vi "move.vi"(10 "dist(mm)":dbl, 11 "Manual Positioning":T1) -> (3 "MoveString":string)   [LabVIEW 2022 SP3]
uses:
  MoveSwitch.ctl
panel:
  out "number":i32
  out "array":bool[](array[boolean])
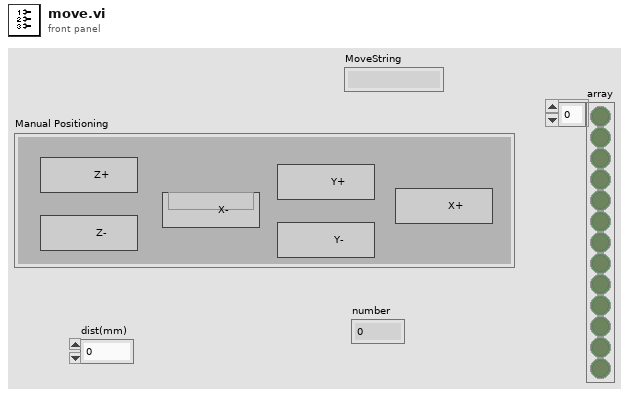
[diagram p1: front panel]
types:
  T1 = typedef "MoveSwitch.ctl" = cluster{"X+":bool, "X-":bool, "Y+":bool, "Y-":bool, "Z+":bool, "Z-":bool}
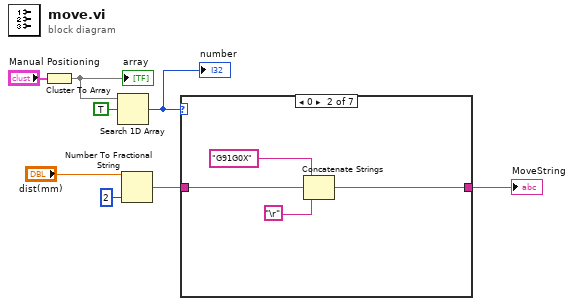
[diagram p0: block diagram]
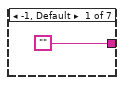
[diagram p2: hidden frame]
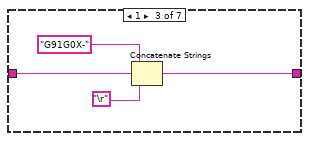
[diagram p3: hidden frame]
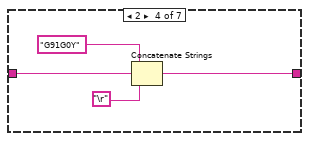
[diagram p4: hidden frame]
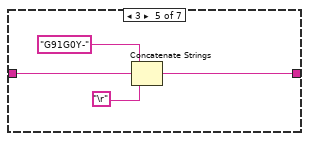
[diagram p5: hidden frame]
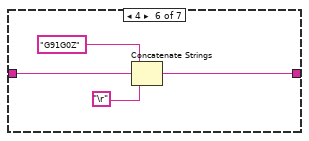
[diagram p6: hidden frame]
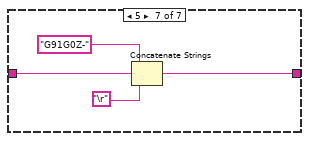
[diagram p7: hidden frame]
diagram:
  n1 = Cluster To Array(cluster="Manual Positioning") -> (array=w7:bool[])
  "array" <- w7
  n2 = Search 1D Array(1D array=w7, element=TRUE) -> (index of element=w5:i32)  [unwired: 1 in]
  "number" <- w5
  n3 = Number To Fractional String(number="dist(mm)", precision (6)=i16 2) -> (F-format string=w2:string)  [unwired: 2 in]
  n4 = case shown="0" w5 {
    tunnel: w2 -> [_ w12 w16 w20 w24 w28 w32]
    tunnel: ["" w10 w14 w18 w22 w26 w30] -> w1
    frame -1, Default {
    }
    frame 0 {
      n5 = Concatenate Strings("G91G0X", w12, "\r") -> (w10:string)
    }
    frame 1 {
      n6 = Concatenate Strings("G91G0X-", w16, "\r") -> (w14:string)
    }
    frame 2 {
      n7 = Concatenate Strings("G91G0Y", w20, "\r") -> (w18:string)
    }
    frame 3 {
      n8 = Concatenate Strings("G91G0Y-", w24, "\r") -> (w22:string)
    }
    frame 4 {
      n9 = Concatenate Strings("G91G0Z", w28, "\r") -> (w26:string)
    }
    frame 5 {
      n10 = Concatenate Strings("G91G0Z-", w32, "\r") -> (w30:string)
    }
  }
  "MoveString" <- w1
